vi "Get Children.vi"(0 "Tree Reference In":refnum<vi>, 2 "Parent Tag":string, 5 "error in (no error)":errorcluster, 9 "Use Current":bool=TRUE) -> (14 "Tree Reference Out":refnum<vi>, 16 "Children Tags":string[](array[string]), 19 "error out":errorcluster)   [LabVIEW 2015, in "QuickVIew.lvlib"]
doc: "Collects and returns all tags of parents immediate children. If the parent tag is an empty string, the currently selected item is used.TLB Prime - Application Template 1.3.0.24\nNorm Kirchner, NI Systems Engineering - NI\nCopyright (c) 2014, NI"
uses:
  QuickVIew.lvlib
panel:
  # "VI INPUTS"
  # "VI OUTPUTS"
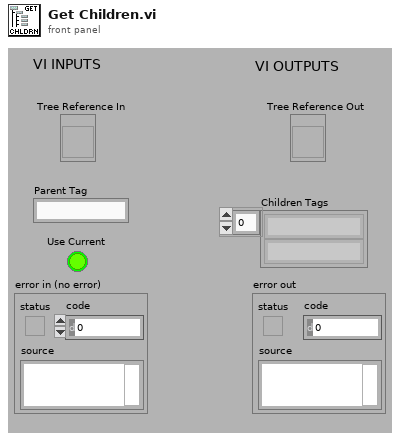
[diagram p1: front panel]
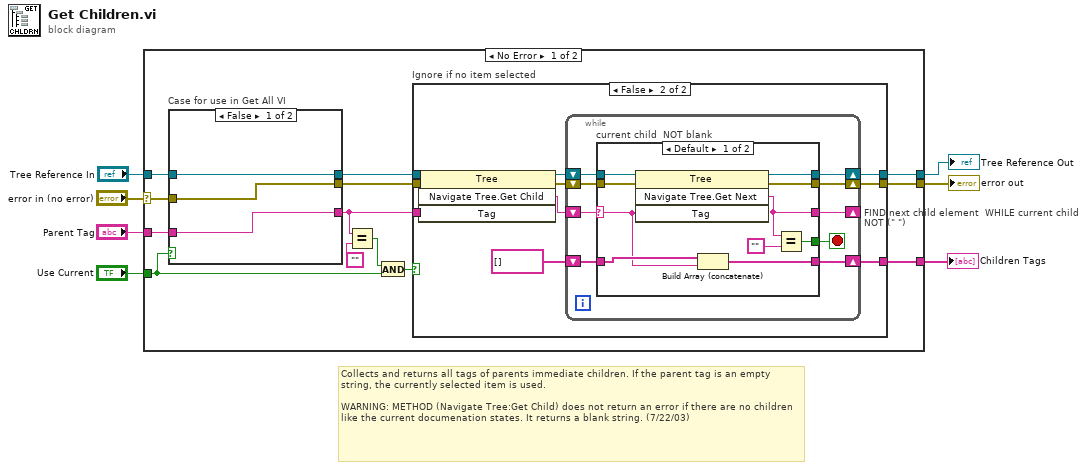
[diagram p0: block diagram]
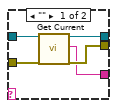
[diagram p3: hidden frame]
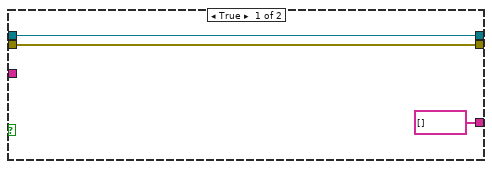
[diagram p4: hidden frame]
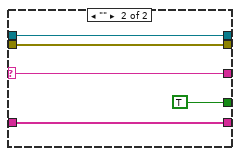
[diagram p5: hidden frame]
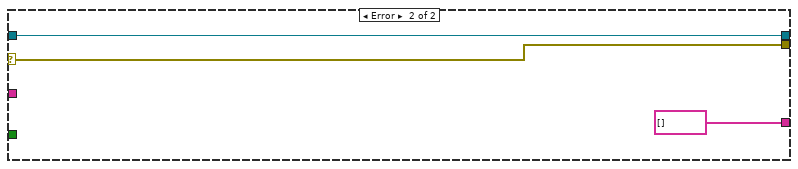
[diagram p6: hidden frame]
diagram:
  # "Collects and returns all tags of parents immediate children. If the parent tag is an empty string, the currently selected item is used. \n\nWARNING: METHOD (Navigate Tree:Get Child) does not return an error if there are no children like the current documenation states. It returns a blank string. (7/22/03)"
  n1 = case shown="No Error" "error in (no error)" {
    selector: "error in (no error)" -> [w15 w76]
    tunnel: "Tree Reference In" -> [w17 w77]
    tunnel: "Parent Tag" -> [w13 _]
    tunnel: [w20 w77] -> w6
    tunnel: [w19 string[] []] -> w5
    tunnel: [w18 w76] -> w4
    tunnel: "Use Current" -> [w9 _]
    frame No Error {
      n2 = case "Case for use in Get All VI" shown="False" w9 {
        tunnel: w17 -> [w23 w29]
        tunnel: [w23 w28] -> w16
        tunnel: w15 -> [w22 w27]
        tunnel: [w22 w26] -> w14
        tunnel: w13 -> [w21 w25]
        tunnel: [w21 w24] -> w12
        frame False {
        }
        frame True {
          n3 = case "Select Current if Empty String" shown="Default" w25 {
            selector: w25 -> [_ w35]
            tunnel: [w33 w37] -> w28
            tunnel: w29 -> [w34 w37]
            tunnel: [w32 w36] -> w26
            tunnel: w27 -> [w31 w36]
            tunnel: [w30 w35] -> w24
            frame "" {
              n4 = call "Get Current.vi"("Tree Reference In"=w34, "error in (no error)"=w31) -> ("Tree Reference Out"=w33:refnum<vi>, "Current Tag"=w30:string, "error out"=w32:errorcluster)  [unwired: 15 out]
            }
            frame Default {
            }
          }
        }
      }
      n5 = Equal?(x=w12, y="") -> (x = y?=w10:bool)
      n6 = And(x=w10, y=w9) -> (x .and. y?=w11:bool)
      n7 = case "Ignore if no item selected" shown="False" w11 {
        tunnel: [w40 w46] -> w20
        tunnel: [string[] [] w45] -> w19
        tunnel: [w39 w44] -> w18
        tunnel: w16 -> [w40 w43]
        tunnel: w14 -> [w39 w42]
        tunnel: w12 -> [_ w41]
        frame True {
        }
        frame False {
          n8 = invoke class="Tree" method="Navigate Tree.Get Child"(reference=w43, error in=w42, "Tag"=w41) -> (reference out=w49:refnum<vi>, error out=w50:errorcluster, "Navigate Tree:Get Child"=w47:string)  [unwired: 1 in, 1 out]
          n9 = while "FIND next child element  WHILE current child  NOT (\" \")" {
            shift-right: [w57] -> w45
            shift-left: string[] [] -> [w56]
            shift-right: [w58] -> w44
            shift-left: w50 -> [w52]
            shift-right: [w54] -> _
            shift-left: w47 -> [w51]
            shift-right: [w53] -> w46
            shift-left: w49 -> [w59]
            stop <- w55 stop-if-true
            n10 = case "current child  NOT blank" shown="Default" w51 {
              selector: w51 -> [w60 w71]
              tunnel: w59 -> [w69 w73]
              tunnel: [w68 w72] -> w58
              tunnel: [w67 w70] -> w57
              tunnel: w56 -> [w66 w70]
              tunnel: [w63 TRUE] -> w55
              tunnel: [w64 w71] -> w54
              tunnel: [w62 w73] -> w53
              tunnel: w52 -> [w61 w72]
              frame Default {
                n11 = invoke class="Tree" method="Navigate Tree.Get Next"(reference=w69, error in=w61, "Tag"=w60) -> (reference out=w62:refnum<vi>, error out=w68:errorcluster, "Navigate Tree:Get Next Item"=w64:string)  [unwired: 1 in, 1 out]
                n12 = Build Array (concatenate)(w66, w60) -> (w67:string[])
                n13 = Equal?(x=w64, y="") -> (x = y?=w63:bool)
              }
              frame "" {
              }
            }
          }
        }
      }
    }
    frame Error {
    }
  }
  "Children Tags" <- w5
  "Tree Reference Out" <- w6
  "error out" <- w4
